vi "Speak.vi"(8 "Error In":errorcluster, 11 "reference in":refnum<class "SpeakTurkish.lvclass">) -> (0 "Error Out":errorcluster, 2 "Result":string, 3 "reference out":refnum<class "SpeakTurkish.lvclass">)   [LabVIEW 2024, in "SpeakTurkish.lvclass"]
uses:
  SpeakTurkish.lvclass
  SpeakTurkish.lvclass/SpeakTurkish.ctl
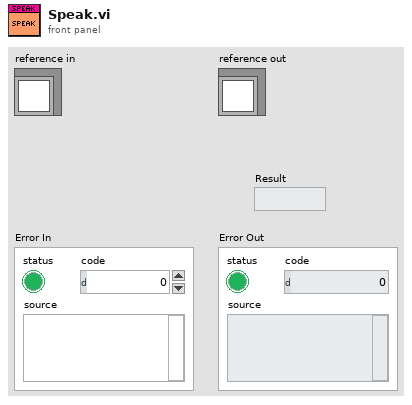
[diagram p1: front panel]
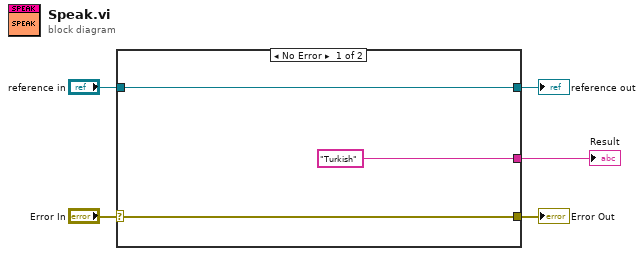
[diagram p0: block diagram]
diagram:
  n1 = case shown="No Error" "Error In" {
    selector: "Error In" -> [w7 w10]
    tunnel: [w7 w10] -> w4
    tunnel: [w8 w9] -> w2
    tunnel: "reference in" -> [w8 w9]
    tunnel: ["Turkish" _] -> w1
    frame No Error {
    }
    frame Error {
    }
  }
  "Error Out" <- w4
  "reference out" <- w2
  "Result" <- w1
